vi "Autonomous Independent.vi"() -> ()   [LabVIEW 2016]
doc: "This VI is called when autonomous begins, and will automatically be terminated when autonomous ends. You can carry out timed or sensor driven robot movement independently without needing to return to the caller."
uses:
  2_8_17/Auto_Action.ctl
  <vilib>/Rock Robotics/Network Tables/NT Read Number.vi
  2_11_17/Systems/Global 1.vi
panel:
  out "Terminated?":bool
  out "Auto Mode":dbl=7.0
  in  "Auton_Modes":T2(array[cluster])=[{"Actions"=[{"Effort"=0.55, "Duration"=3.5, "Action"=enum."Nothing", "Encoder"=0.0, "Condition"=FALSE}, {"Effort"=0.0, "Duration"=0.0, "Action"=enum."Nothing", "Encoder"=0.0, "Condition"=FALSE}]}, {"Actions"=[{"Effort"=0.0, "Duration"=0.1, "Action"=enum."Gear1", "Encoder"=6.462, "Condition"=FALSE}, {"Effort"=0.0, "Duration"=0.1, "Action"=enum."Nothing", "Encoder"=0.0, "Condition"=FALSE}, {"Effort"=0.25, "Duration"=1.0, "Action"=enum."Nothing", "Encoder"=38.0, "Condition"=FALSE}, {"Effort"=0.0, "Duration"=0.1, "Action"=enum."Nothing", "Encoder"=0.0, "Condition"=FALSE}, {"Effort"=0.25, "Duration"=0.0, "Action"=enum."Nothing", "Encoder"=57.0, "Condition"=FALSE}, {"Effort"=-0.25, "Duration"=0.0, "Action"=enum."Nothing", "Encoder"=0.0, "Condition"=FALSE}, {"Effort"=1.0, "Duration"=0.0, "Action"=enum."Nothing", "Encoder"=0.0, "Condition"=FALSE}, {"Effort"=0.25, "Duration"=0.0, "Action"=enum."Nothing", "Encoder"=0.0, "Condition"=FALSE}]}, {"Actions"=[{"Effort"=0.0, "Duration"=0.1, "Action"=enum."Drive Encoder Reset", "Encoder"=0.0, "Condition"=FALSE}, {"Effort"=0.0, "Duration"=1.0, "Action"=enum."Gyro Reset", "Encoder"=0.0, "Condition"=FALSE}, {"Effort"=500.0, "Duration"=3.5, "Action"=enum."Drive", "Encoder"=88.0, "Condition"=FALSE}, {"Effort"=1.0, "Duration"=1.0, "Action"=enum."Gear0", "Encoder"=0.0, "Condition"=FALSE}, {"Effort"=1.0, "Duration"=1.0, "Action"=enum."Gear0", "Encoder"=0.0, "Condition"=FALSE}, {"Effort"=1.0, "Duration"=0.5, "Action"=enum."Nothing", "Encoder"=0.0, "Condition"=FALSE}, {"Effort"=0.0, "Duration"=0.0, "Action"=enum."Drive Encoder Reset", "Encoder"=0.0, "Condition"=FALSE}, {"Effort"=500.0, "Duration"=0.5, "Action"=enum."Drive", "Encoder"=24.0, "Condition"=TRUE}, {"Effort"=0.0, "Duration"=0.0, "Action"=enum."Drive Encoder Reset", "Encoder"=0.0, "Condition"=FALSE}, {"Effort"=-500.0, "Duration"=0.0, "Action"=enum."Drive", "Encoder"=24.0, "Condition"=FALSE}, {"Effort"=0.0, "Duration"=0.0, "Action"=enum."Drive Encoder Reset", "Encoder"=0.0, "Condition"=FALSE}, {"Effort"=-0.25, "Duration"=0.0, "Action"=enum."Nothing", "Encoder"=12.0, "Condition"=FALSE}]}, {"Actions"=[{"Effort"=0.0, "Duration"=0.1, "Action"=enum."Drive Encoder Reset", "Encoder"=6.462, "Condition"=FALSE}, {"Effort"=0.0, "Duration"=0.1, "Action"=enum."Gyro Reset", "Encoder"=0.0, "Condition"=FALSE}, {"Effort"=-0.25, "Duration"=1.0, "Action"=enum."Drive", "Encoder"=6.462, "Condition"=FALSE}, {"Effort"=0.0, "Duration"=0.1, "Action"=enum."Gyro Reset", "Encoder"=0.0, "Condition"=FALSE}, {"Effort"=-0.25, "Duration"=0.0, "Action"=enum."Turn", "Encoder"=57.0, "Condition"=FALSE}, {"Effort"=-0.25, "Duration"=0.0, "Action"=enum."Drive", "Encoder"=7.5, "Condition"=FALSE}, {"Effort"=-1.0, "Duration"=0.0, "Action"=enum."Gear0", "Encoder"=0.0, "Condition"=FALSE}, {"Effort"=0.25, "Duration"=0.0, "Action"=enum."Drive", "Encoder"=3.0, "Condition"=FALSE}]}, {"Actions"=[{"Effort"=0.0, "Duration"=0.1, "Action"=enum."Drive Encoder Reset", "Encoder"=6.462, "Condition"=FALSE}, {"Effort"=0.0, "Duration"=0.1, "Action"=enum."Gyro Reset", "Encoder"=0.0, "Condition"=FALSE}, {"Effort"=-0.25, "Duration"=1.0, "Action"=enum."Drive", "Encoder"=6.462, "Condition"=FALSE}, {"Effort"=0.0, "Duration"=0.1, "Action"=enum."Gyro Reset", "Encoder"=0.0, "Condition"=FALSE}, {"Effort"=-0.25, "Duration"=0.0, "Action"=enum."Turn", "Encoder"=57.0, "Condition"=FALSE}, {"Effort"=-0.25, "Duration"=0.0, "Action"=enum."Drive", "Encoder"=7.5, "Condition"=FALSE}, {"Effort"=-1.0, "Duration"=0.0, "Action"=enum."Gear0", "Encoder"=0.0, "Condition"=FALSE}, {"Effort"=0.25, "Duration"=0.0, "Action"=enum."Drive", "Encoder"=3.0, "Condition"=FALSE}]}, {"Actions"=[{"Effort"=0.0, "Duration"=0.1, "Action"=enum."Drive Encoder Reset", "Encoder"=0.0, "Condition"=FALSE}, {"Effort"=0.0, "Duration"=0.1, "Action"=enum."Gyro Reset", "Encoder"=0.0, "Condition"=FALSE}, {"Effort"=0.25, "Duration"=1.0, "Action"=enum."Drive", "Encoder"=6.462, "Condition"=FALSE}, {"Effort"=1.0, "Duration"=0.1, "Action"=enum."Gyro Reset", "Encoder"=0.0, "Condition"=FALSE}, {"Effort"=0.25, "Duration"=0.0, "Action"=enum."Turn", "Encoder"=57.0, "Condition"=FALSE}, {"Effort"=0.25, "Duration"=0.0, "Action"=enum."Drive", "Encoder"=7.5, "Condition"=FALSE}, {"Effort"=1.0, "Duration"=0.0, "Action"=enum."Gear0", "Encoder"=0.0, "Condition"=FALSE}, {"Effort"=-0.25, "Duration"=0.0, "Action"=enum."Drive", "Encoder"=3.0, "Condition"=FALSE}]}, {"Actions"=[{"Effort"=0.0, "Duration"=0.1, "Action"=enum."Drive Encoder Reset", "Encoder"=0.0, "Condition"=FALSE}, {"Effort"=0.0, "Duration"=0.1, "Action"=enum."Gyro Reset", "Encoder"=0.0, "Condition"=FALSE}, {"Effort"=0.25, "Duration"=2.0, "Action"=enum."Drive", "Encoder"=60.0, "Condition"=FALSE}, {"Effort"=0.75, "Duration"=1.0, "Action"=enum."Nothing", "Encoder"=0.0, "Condition"=FALSE}, {"Effort"=0.0, "Duration"=1.0, "Action"=enum."Nothing", "Encoder"=0.0, "Condition"=FALSE}, {"Effort"=0.0, "Duration"=0.0, "Action"=enum."Nothing", "Encoder"=0.0, "Condition"=FALSE}]}, {"Actions"=[{"Effort"=0.0, "Duration"=0.5, "Action"=enum."Drive Encoder Reset", "Encoder"=0.0, "Condition"=FALSE}, {"Effort"=0.55, "Duration"=4.25, "Action"=enum."Gyro Reset", "Encoder"=0.0, "Condition"=FALSE}, {"Effort"=500.0, "Duration"=0.0, "Action"=enum."Drive", "Encoder"=60.0, "Condition"=FALSE}, {"Effort"=0.25, "Duration"=1.4, "Action"=enum."Turn", "Encoder"=0.0, "Condition"=FALSE}, {"Effort"=0.25, "Duration"=2.0, "Action"=enum."Vision Correction", "Encoder"=76.6, "Condition"=FALSE}, {"Effort"=500.0, "Duration"=0.0, "Action"=enum."Drive", "Encoder"=0.0, "Condition"=FALSE}]}, {"Actions"=[{"Effort"=0.0, "Duration"=0.0, "Action"=enum."Nothing", "Encoder"=0.0, "Condition"=FALSE}]}]
  # "Nothing"
  # "Boiler Right Right side gear"
  # "Middle Gear"
  # "Boiler Right Left Side Gear"
  # "Boiler Left RightSide Gear"
  # "Boiler Left Left Side Gear"
  # "Drive"
  # "Vision Correction"
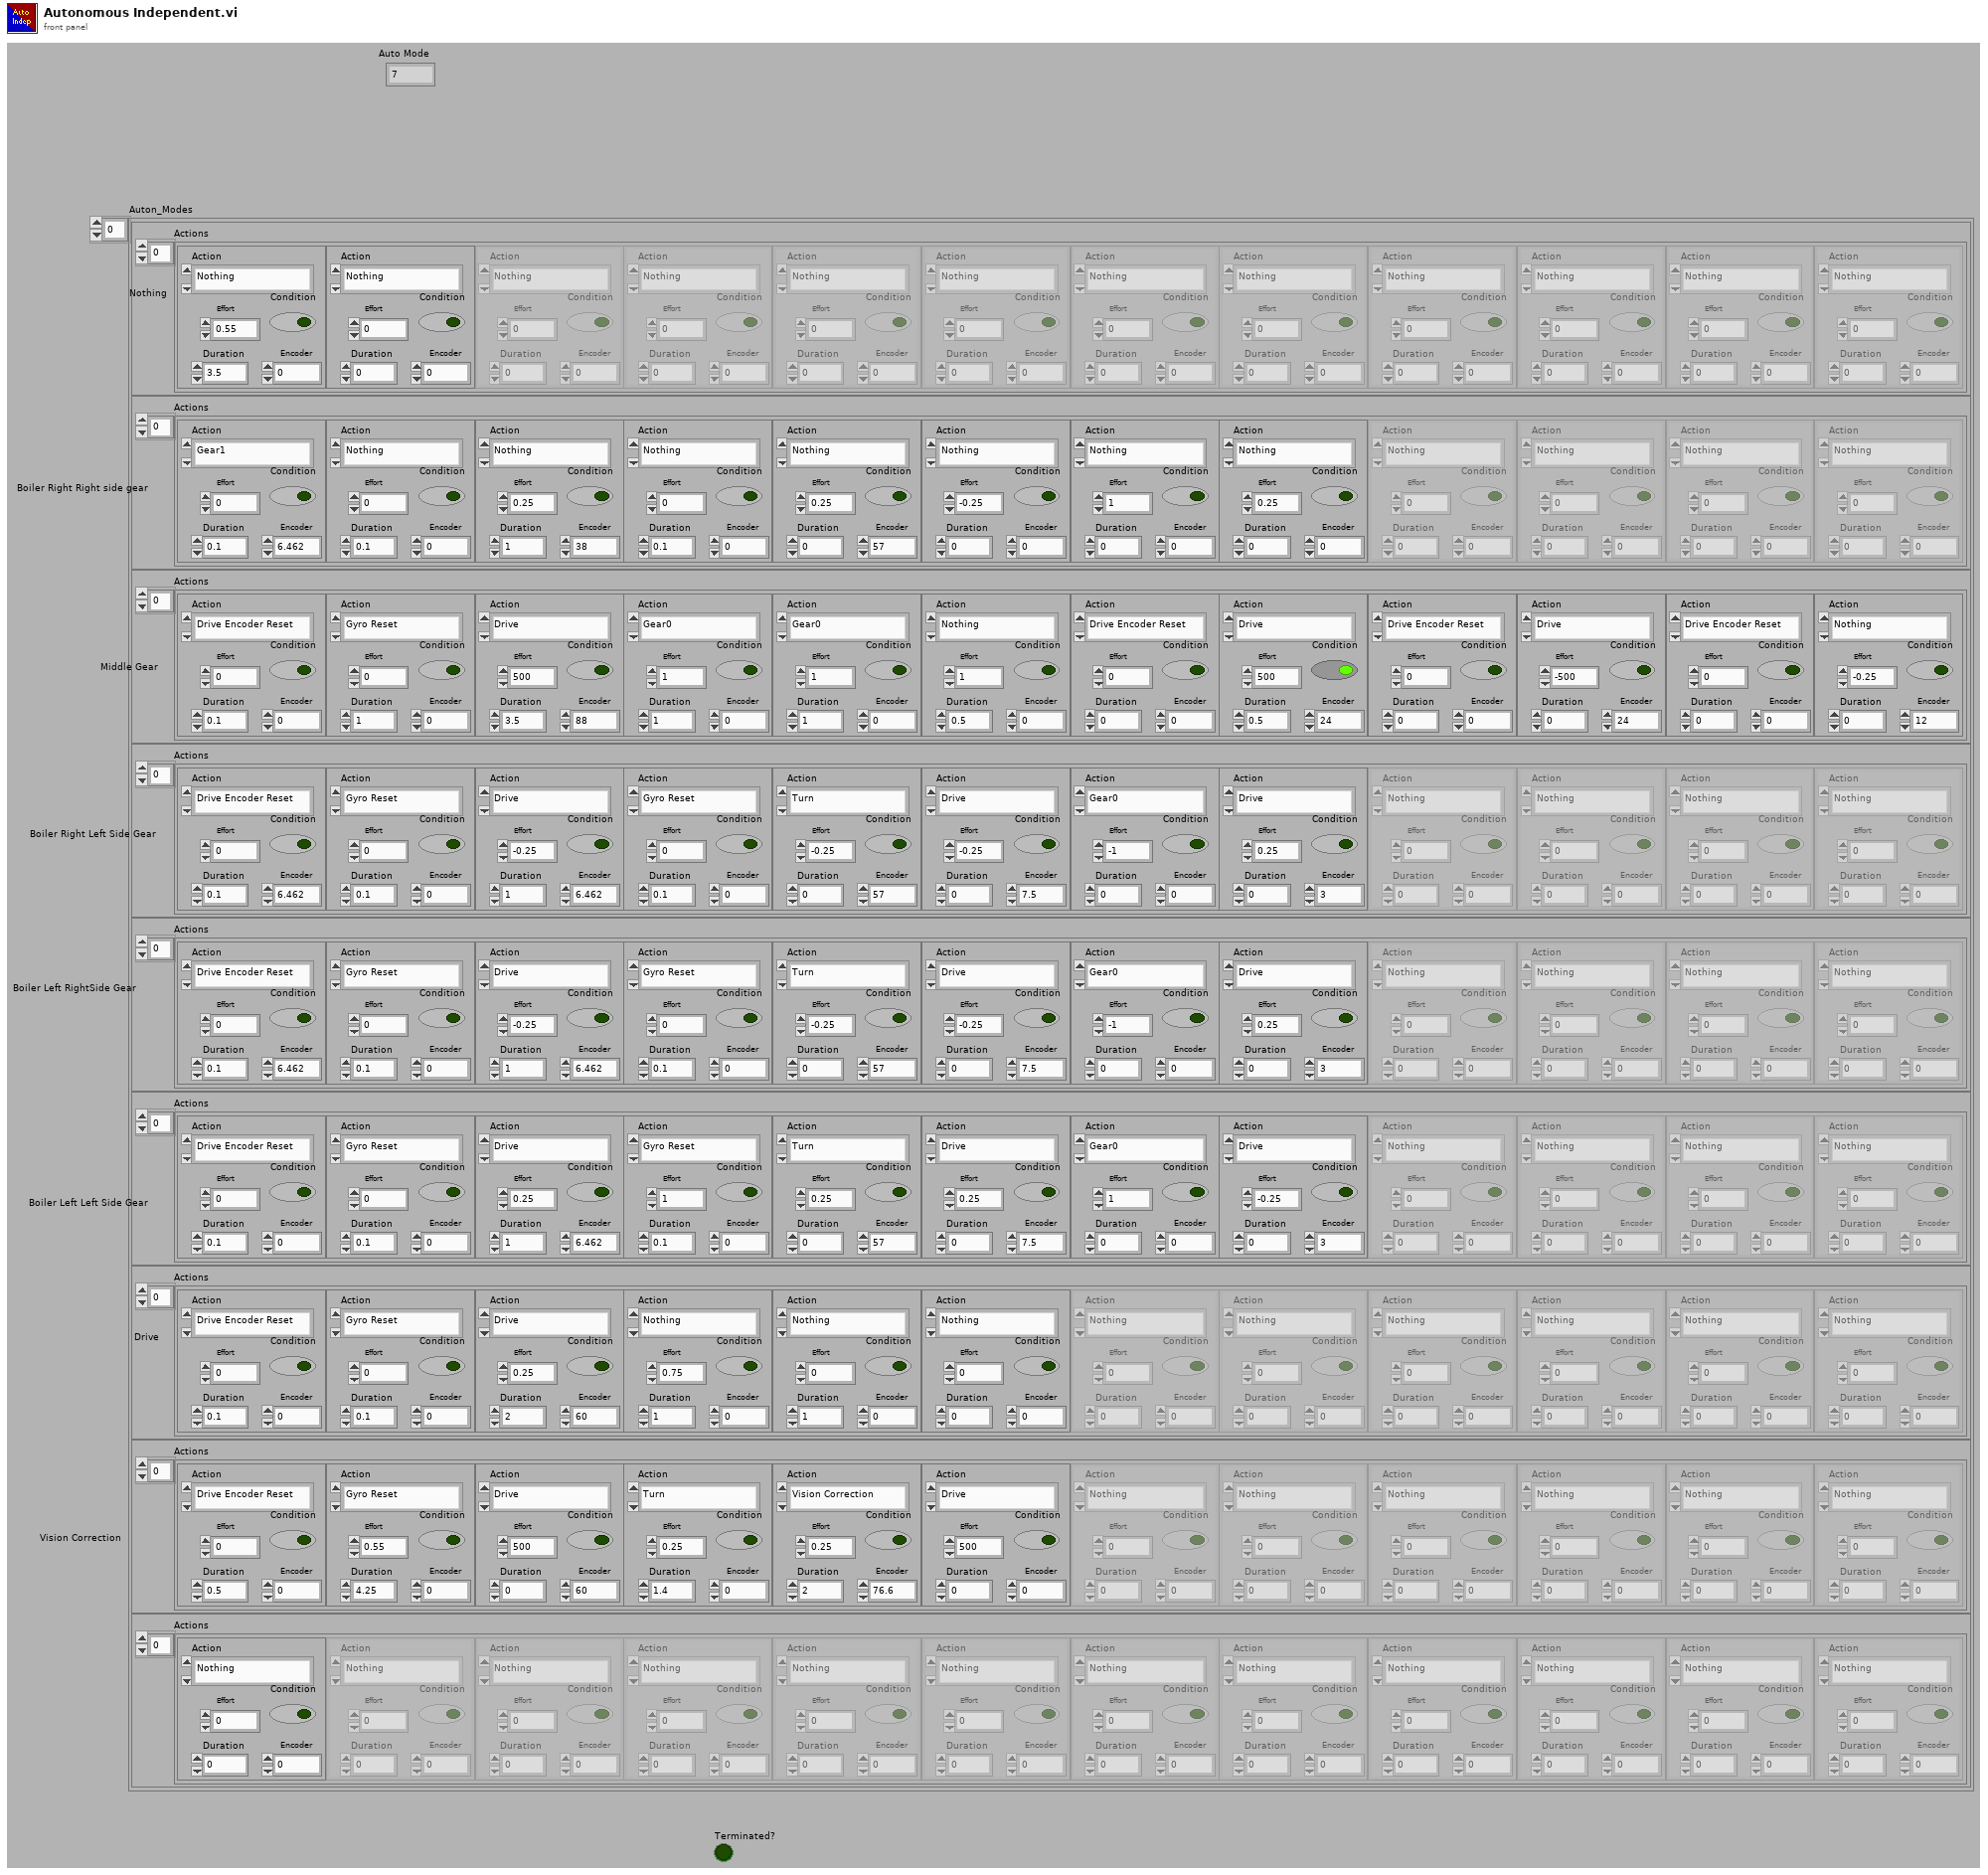
[diagram p1: front panel]
types:
  T1 = typedef "Auto_Action.ctl" = enum16{"Nothing", "Drive", "Vision Correction", "Turn", "Gear0", "Gear1", "Climb", "Intake", "Index", "Shoot", "Test", "Drive Encoder Reset", "Gyro Reset"}
  T2 = cluster{"Actions":cluster{"Effort":dbl, "Duration":dbl, "Action":T1, "Encoder":dbl, "Condition":bool}[]}[]
  T3 = cluster{"Actions":cluster{"Effort":dbl, "Duration":dbl, "Action":T1, "Encoder":dbl, "Condition":bool}[]}
  T4 = cluster{"Effort":dbl, "Duration":dbl, "Action":T1, "Encoder":dbl, "Condition":bool}[]
  T5 = typedef "WPI_MotorControlDeviceRef.ctl" = cluster{"DeviceStatus":errorcluster, "Type":T6, "PWM":cluster{"PWM Channel":T7, "DeadBand":T8}, "CAN":cluster{"Device Number":u8, "SetOutput VI Ref":variant, "GetOutput VI Ref":variant, "Enable VI Ref":variant, "Disable VI Ref":variant, "Data":variant}, "Invert":bool}
  T6 = typedef "WPI_MotorControlType.ctl" = enum16{"PWM", "CAN"}
  T7 = typedef "FPGA_DIOPWMChannel.ctl" = enum8{"PWM 0", "PWM 1", "PWM 2", "PWM 3", "PWM 4", "PWM 5", "PWM 6", "PWM 7", "PWM 8", "PWM 9", "PWM MXP 0", "PWM MXP 1", "PWM MXP 2", "PWM MXP 3", "PWM MXP 4", "PWM MXP 5", "PWM MXP 6", "PWM MXP 7", "PWM MXP 8", "PWM MXP 9", "Invalid"}
  T8 = typedef "WPI_PWMDeadband.ctl" = cluster{"Name":string, "maxPositivePwm":i32, "minPositivePwm":i32, "centerPwm":i32, "maxNegativePwm":i32, "minNegativePwm":i32, "angularRange":u16}
  T9 = typedef "WPI_CANTalonSRX_GlobalStatus.ctl" = cluster{"Applied Throttle":dbl, "Module Enabled":bool, "CAN Error":errorcluster, "Closed Loop Error":dbl, "Forward Limit Switch Closed":bool, "Reverse Limit Switch Closed":bool, "Sensor Position":dbl, "Sensor Velocity":dbl, "Current":dbl, "Sticky Fault - Over Temp":bool, "Sticky Fault - Under Voltage":bool, "Sticky Fault - Forward Limit":bool, "Sticky Fault - Reverse Limit":bool, "Sticky Fault - Forward Soft Limit":bool, "Sticky Fault - Reverse Soft Limit":bool, "Brake is Enabled":bool, "Encoder Position":dbl, "Encoder Velocity":dbl, "Encoder Index Count":dbl, "Encoder A Pin State":bool, "Encoder B Pin State":bool, "Encoder Index Pin State":bool, "Analog In":dbl, "Analog In Velocity":dbl, "Temperature (C)":dbl, "Battery Voltage":dbl, "Control 5 Is Supported":bool, "Current Profile Slot Select":dbl, "Pos Div 8":bool, "Vel Div 4":bool, "Pulse Width Position":i32, "Pulse Width Velocity":i32, "Pulse Width Rise To Rise (us)":i32, "Pulse Width Rise To Fall (us)":i32, "Mot Prof Active Is Under Run":bool, "Mot Prof Active Has Under Run":bool, "Mot Prof Active Is Last":bool, "Mot Prof Active Velocity Only":bool, "Mot Prof Active Is Valid":bool, "Mot Prof Buffer Is Full":bool, "Mot Prof Active Profile Slot Select":i32, "Mot Prof NextID":i32, "Mot Prof Count":i32, "Mot Prof Active Velocity":dbl, "Mot Prof Active Position":dbl, "Mot Prof Output Enable":i32}
  T10 = typedef "WPI_GyroDevRef.ctl" = cluster{"DevStatus":errorcluster, "Analog Channel":T11, "Offset":dbl, "Gain (VoltsPerDegree/Second)":dbl, "Gyro Type":enum16{"Analog", "XRS450"}, "Handle":i32, "SPI Bus":T12, "Device Found":bool, "Sample Rate":dbl, "Calibrate On Open":bool}
  T11 = typedef "FPGA_AIChannel.ctl" = enum8{"AI 0", "AI 1", "AI 2", "AI 3", "AI MXP 0", "AI MXP 1", "AI MXP 2", "AI MXP 3", "Invalid"}
  T12 = typedef "spi_bus.ctl" = enum16{"SPI On-Board, CS0", "SPI On-Board, CS1", "SPI On-Board, CS2", "SPI On-Board, CS3", "SPI MXP", "Invalid"}
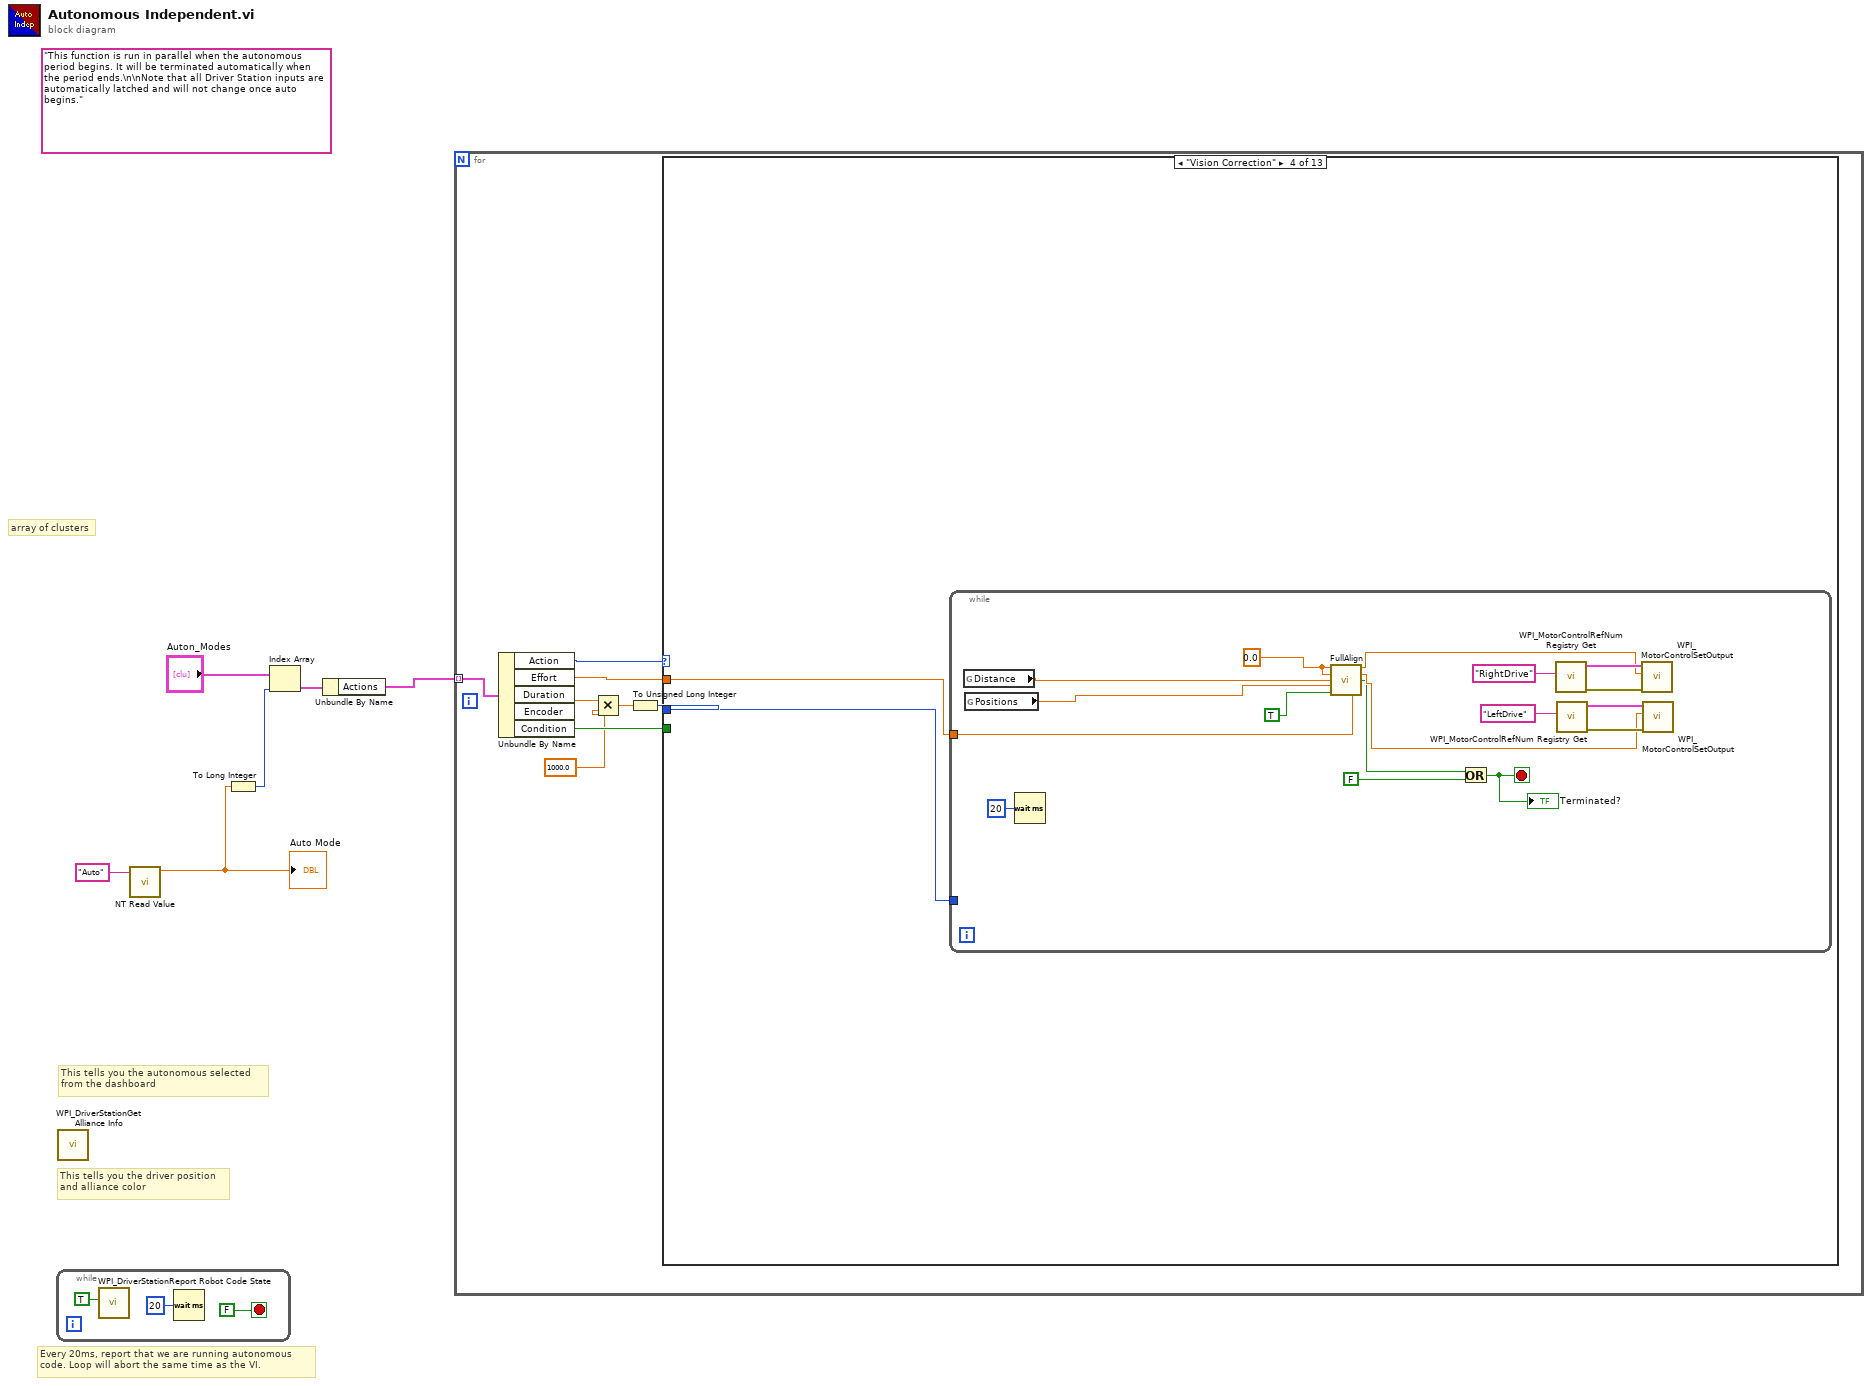
[diagram p0: block diagram]
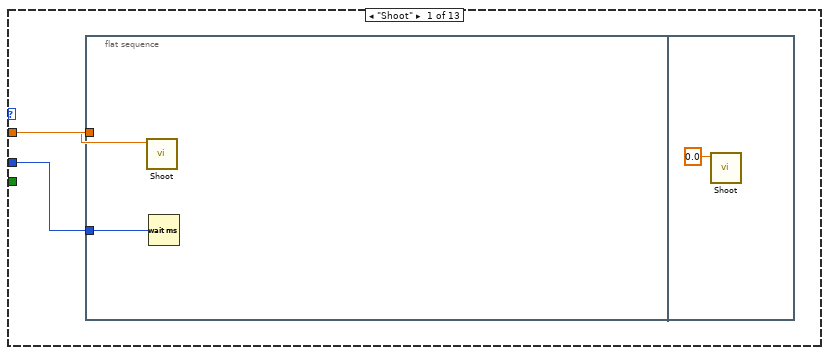
[diagram p2: hidden frame]
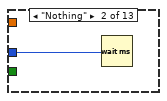
[diagram p3: hidden frame]
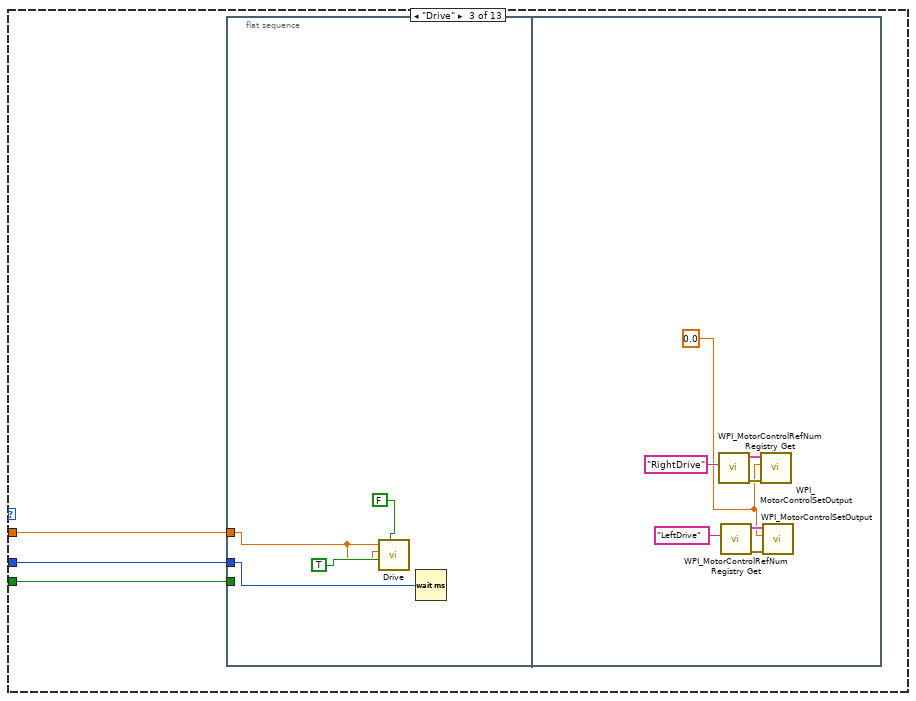
[diagram p4: hidden frame]
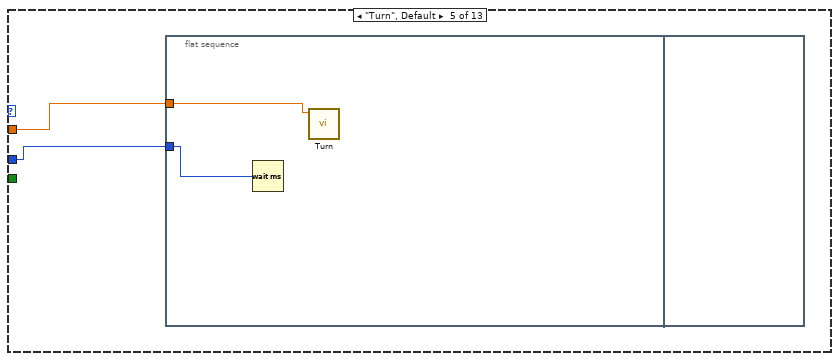
[diagram p5: hidden frame]
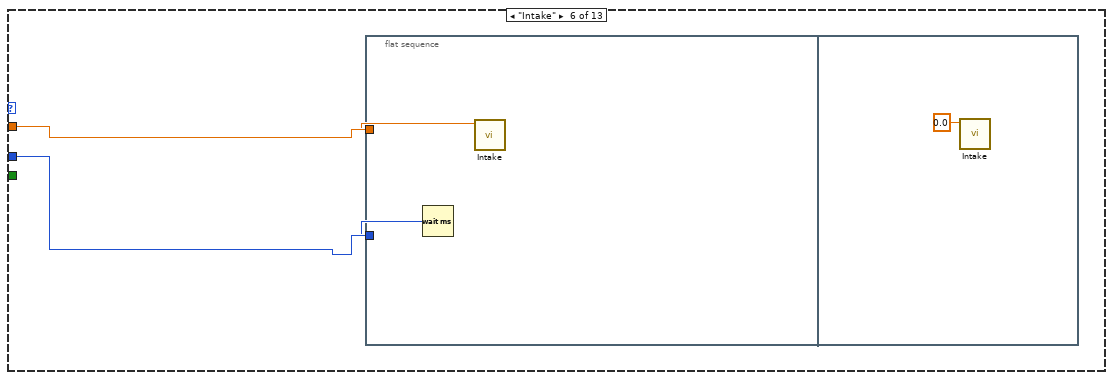
[diagram p6: hidden frame]
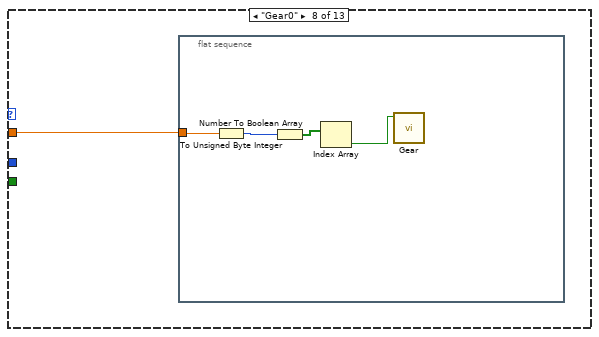
[diagram p8: hidden frame]
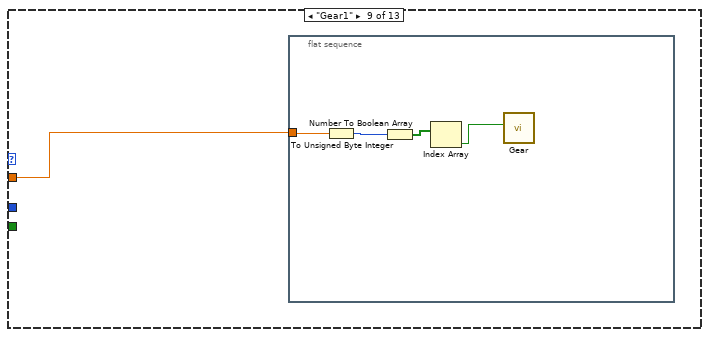
[diagram p9: hidden frame]
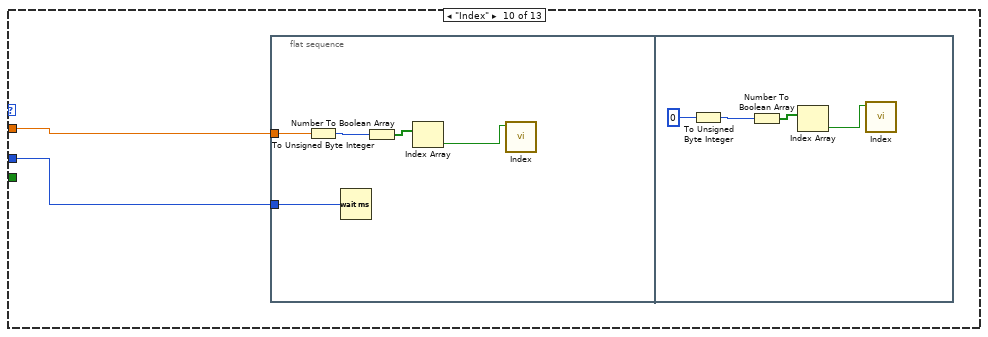
[diagram p10: hidden frame]
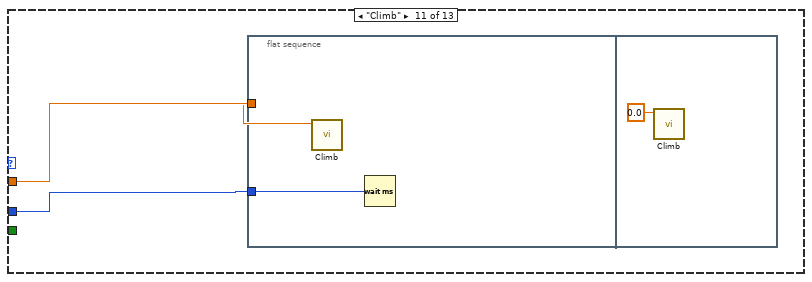
[diagram p11: hidden frame]
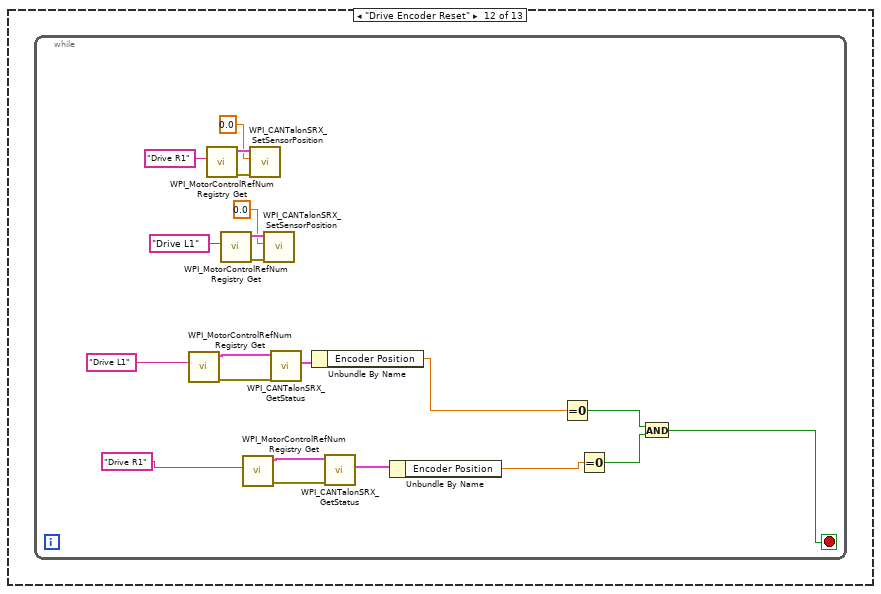
[diagram p12: hidden frame]
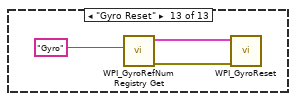
[diagram p13: hidden frame]
diagram:
  (unwired) "This function is run in parallel when the autonomous period begins. It will be terminated automatically when the period ends.\n\nNote that all Driver Station inputs are automatically latched and will not change once auto begins."
  # "This tells you the autonomous selected\nfrom the dashboard"
  # "array of clusters"
  # "Every 20ms, report that we are running autonomous\ncode. Loop will abort the same time as the VI."
  # "This tells you the driver position\nand alliance color"
  n1 = while {
    stop <- FALSE stop-if-true
    n2 = call <vilib>:"WPI_DriverStationReport Robot Code State.vi"("Autonomous"=TRUE) -> ()  [unwired: 10 in, 1 out]
    n3 = Wait (ms)(milliseconds to wait=u32 20) -> ()  [unwired: 1 out]
  }
  n4 = call <vilib>:"WPI_DriverStationGet Alliance Info.vi"() -> ()  [unwired: 12 out]
  n5 = call-poly <vilib>:"NT Read Value.vi"("Name"="Auto") -> ("Numeric"=w1:dbl)  [unwired: 9 in, 1 out]
  "Auto Mode" <- w1
  n6 = To Long Integer(number=w1) -> (32bit integer=w3:i32)
  n7 = Index Array(array="Auton_Modes", index=w3) -> (element=w5:T3)
  n8 = Unbundle By Name(w5) -> ("Actions"=w6:T4)
  n9 = for {
    tunnel: w6 -> [w17] mode=indexing
    n10 = Unbundle By Name(w17) -> ("Action"=w16:T1, "Effort"=w15:dbl, "Duration"=w14:dbl, "Condition"=w11:bool)  [unwired: 1 out]
    n11 = Multiply(x=w14, y=1000.0) -> (x*y=w13:dbl)
    n12 = To Unsigned Long Integer(number=w13) -> (unsigned 32bit integer=w12:u32)
    n13 = case shown="\"Vision Correction\"" w16 {
      tunnel: w15 -> [w19 _ w26 w38 w58 w62 _ w66 w71 w76 w88 _ _]
      tunnel: w12 -> [w18 w23 w25 w39 w57 w61 _ _ _ w77 w87 _ _]
      tunnel: w11 -> [_ _ w24 _ _ _ _ _ _ _ _ _ _]
      frame "Shoot" {
        n14 = flat-sequence {
          tunnel: w19 -> [w21]
          tunnel: w18 -> [w20]
          frame #0 {
            n15 = call "Shoot.vi"("Set RPM"=w21) -> ()  [unwired: 11 in]
            n16 = Wait (ms)(milliseconds to wait=w20) -> ()  [unwired: 1 out]
          }
          frame #1 {
            n17 = call "Shoot.vi"("Set RPM"=0.0 ("Effort")) -> ()  [unwired: 11 in]
          }
        }
      }
      frame "Nothing" {
        n18 = Wait (ms)(milliseconds to wait=w23) -> ()  [unwired: 1 out]
      }
      frame "Drive" {
        n19 = flat-sequence {
          tunnel: w26 -> [w27]
          tunnel: w25 -> [w30]
          tunnel: w24 -> [_]
          frame #0 {
            n20 = call "Drive.vi"("Slow?"=FALSE, "SwitchDir"=TRUE, "Drive L"=w27, "Drive R"=w27) -> ()  [unwired: 8 in]
            n21 = Wait (ms)(milliseconds to wait=w30) -> ()  [unwired: 1 out]
          }
          frame #1 {
            w31 = 0.0
            n22 = call <vilib>:"WPI_MotorControlRefNum Registry Get.vi"("refnum name"="RightDrive") -> ("error out"=w34:errorcluster, "MotorControlDevRef"=w32:T5)  [unwired: 9 in]
            n23 = call <vilib>:"WPI_MotorControlRefNum Registry Get.vi"("refnum name"="LeftDrive") -> ("error out"=w35:errorcluster, "MotorControlDevRef"=w36:T5)  [unwired: 9 in]
            n24 = call <vilib>:"WPI_MotorControlSetOutput.vi"("error in (no error)"=w34, "Output"=w31, "MotorControlDevRef"=w32) -> ()  [unwired: 6 in, 3 out]
            n25 = call <vilib>:"WPI_MotorControlSetOutput.vi"("error in (no error)"=w35, "Output"=w31, "MotorControlDevRef"=w36) -> ()  [unwired: 6 in, 3 out]
          }
        }
      }
      frame "Vision Correction" {
        n26 = while {
          tunnel: w39 -> [_]
          tunnel: w38 -> [w40]
          stop <- w44 stop-if-true
          w48 = 0.0
          n27 = global read "Global 1.vi" "Distance"() -> (w46:dbl)
          n28 = global read "Global 1.vi" "Positions"() -> (w45:dbl)
          n29 = Wait (ms)(milliseconds to wait=u32 20) -> ()  [unwired: 1 out]
          n30 = call "FullAlign.vi"("Joystick 0"=w48, "Joystick 1"=w48, "Distance"=w46, "Angle"=w45, "Button"=TRUE, "Effort"=w40) -> ("Right Motor"=w50:dbl, "Left Motor"=w49:dbl, "In Range?"=w42:bool)  [unwired: 6 in, 1 out]
          n31 = Or(x=w42, y=FALSE) -> (x .or. y?=w44:bool)
          "Terminated?" <- w44
          n32 = call <vilib>:"WPI_MotorControlRefNum Registry Get.vi"("refnum name"="RightDrive") -> ("error out"=w51:errorcluster, "MotorControlDevRef"=w53:T5)  [unwired: 9 in]
          n33 = call <vilib>:"WPI_MotorControlRefNum Registry Get.vi"("refnum name"="LeftDrive") -> ("error out"=w54:errorcluster, "MotorControlDevRef"=w55:T5)  [unwired: 9 in]
          n34 = call <vilib>:"WPI_MotorControlSetOutput.vi"("error in (no error)"=w51, "Output"=w50, "MotorControlDevRef"=w53) -> ()  [unwired: 6 in, 3 out]
          n35 = call <vilib>:"WPI_MotorControlSetOutput.vi"("error in (no error)"=w54, "Output"=w49, "MotorControlDevRef"=w55) -> ()  [unwired: 6 in, 3 out]
        }
      }
      frame "Turn", Default {
        n36 = flat-sequence {
          tunnel: w58 -> [w60]
          tunnel: w57 -> [w59]
          frame #0 {
            n37 = Wait (ms)(milliseconds to wait=w59) -> ()  [unwired: 1 out]
            n38 = call "Turn.vi"("Effort"=w60) -> ()  [unwired: 11 in]
          }
          frame #1 {
          }
        }
      }
      frame "Intake" {
        n39 = flat-sequence {
          tunnel: w62 -> [w64]
          tunnel: w61 -> [w63]
          frame #0 {
            n40 = Wait (ms)(milliseconds to wait=w63) -> ()  [unwired: 1 out]
            n41 = call "Intake.vi"("Effort"=w64) -> ()  [unwired: 11 in]
          }
          frame #1 {
            n42 = call "Intake.vi"("Effort"=0.0) -> ()  [unwired: 11 in]
          }
        }
      }
      frame "Test" {
      }
      frame "Gear0" {
        n43 = flat-sequence {
          tunnel: w66 -> [w70]
          frame #0 {
            n44 = To Unsigned Byte Integer(number=w70) -> (unsigned 8bit integer=w69:u8)
            n45 = Number To Boolean Array(number=w69) -> (Boolean array=w68:bool[])
            n46 = Index Array(array=w68) -> (element=w67:bool)  [unwired: 1 in]
            n47 = call "Gear.vi"("Gear0?"=w67) -> ()  [unwired: 11 in]
          }
        }
      }
      frame "Gear1" {
        n48 = flat-sequence {
          tunnel: w71 -> [w75]
          frame #0 {
            n49 = To Unsigned Byte Integer(number=w75) -> (unsigned 8bit integer=w74:u8)
            n50 = Number To Boolean Array(number=w74) -> (Boolean array=w73:bool[])
            n51 = Index Array(array=w73) -> (element=w72:bool)  [unwired: 1 in]
            n52 = call "Gear.vi"("Gear1?"=w72) -> ()  [unwired: 11 in]
          }
        }
      }
      frame "Index" {
        n53 = flat-sequence {
          tunnel: w77 -> [w79]
          tunnel: w76 -> [w78]
          frame #0 {
            n54 = To Unsigned Byte Integer(number=w78) -> (unsigned 8bit integer=w82:u8)
            n55 = Wait (ms)(milliseconds to wait=w79) -> ()  [unwired: 1 out]
            n56 = Number To Boolean Array(number=w82) -> (Boolean array=w81:bool[])
            n57 = Index Array(array=w81) -> (element=w80:bool)  [unwired: 1 in]
            n58 = call "Index.vi"("Index?"=w80) -> ()  [unwired: 11 in]
          }
          frame #1 {
            n59 = To Unsigned Byte Integer(number=u8 0) -> (unsigned 8bit integer=w85:u8)
            n60 = Number To Boolean Array(number=w85) -> (Boolean array=w86:bool[])
            n61 = Index Array(array=w86) -> (element=w83:bool)  [unwired: 1 in]
            n62 = call "Index.vi"("Index?"=w83) -> ()  [unwired: 11 in]
          }
        }
      }
      frame "Climb" {
        n63 = flat-sequence {
          tunnel: w88 -> [w90]
          tunnel: w87 -> [w89]
          frame #0 {
            n64 = call "Climb.vi"("Effort"=w90) -> ()  [unwired: 11 in]
            n65 = Wait (ms)(milliseconds to wait=w89) -> ()  [unwired: 1 out]
          }
          frame #1 {
            n66 = call "Climb.vi"("Effort"=0.0) -> ()  [unwired: 11 in]
          }
        }
      }
      frame "Drive Encoder Reset" {
        n67 = while {
          stop <- w92 stop-if-true
          n68 = call <vilib>:"WPI_MotorControlRefNum Registry Get.vi"("refnum name"="Drive L1") -> ("error out"=w102:errorcluster, "MotorControlDevRef"=w97:T5)  [unwired: 9 in]
          n69 = call <vilib>:"WPI_MotorControlRefNum Registry Get.vi"("refnum name"="Drive R1") -> ("error out"=w107:errorcluster, "MotorControlDevRef"=w106:T5)  [unwired: 9 in]
          n70 = call <vilib>:"WPI_MotorControlRefNum Registry Get.vi"("refnum name"="Drive L1") -> ("error out"=w109:errorcluster, "MotorControlDevRef"=w110:T5)  [unwired: 9 in]
          n71 = call <vilib>:"WPI_MotorControlRefNum Registry Get.vi"("refnum name"="Drive R1") -> ("error out"=w99:errorcluster, "MotorControlDevRef"=w98:T5)  [unwired: 9 in]
          n72 = call <vilib>:"WPI_CANTalonSRX_SetSensorPosition.vi"("error in (no error)"=w107, "New Sensor Position"=0.0, "CAN Talon SRX Ref"=w106) -> ()  [unwired: 7 in, 2 out]
          n73 = call <vilib>:"WPI_CANTalonSRX_SetSensorPosition.vi"("error in (no error)"=w109, "New Sensor Position"=0.0, "CAN Talon SRX Ref"=w110) -> ()  [unwired: 7 in, 2 out]
          n74 = call <vilib>:"WPI_CANTalonSRX_GetStatus.vi"("error in (no error)"=w102, "CAN Talon SRX Ref"=w97) -> ("Talon SRX Status"=w100:T9)  [unwired: 7 in, 2 out]
          n75 = Unbundle By Name(w100) -> ("Encoder Position"=w95:dbl)
          n76 = call <vilib>:"WPI_CANTalonSRX_GetStatus.vi"("error in (no error)"=w99, "CAN Talon SRX Ref"=w98) -> ("Talon SRX Status"=w101:T9)  [unwired: 7 in, 2 out]
          n77 = Unbundle By Name(w101) -> ("Encoder Position"=w96:dbl)
          n78 = Equal To 0?(x=w95) -> (x = 0?=w94:bool)
          n79 = Equal To 0?(x=w96) -> (x = 0?=w93:bool)
          n80 = And(x=w94, y=w93) -> (x .and. y?=w92:bool)
        }
      }
      frame "Gyro Reset" {
        n81 = call <vilib>:"WPI_GyroRefNum Registry Get.vi"("refnum name"="Gyro") -> ("error out"=w114:errorcluster, "GyroDevRef"=w115:T10)  [unwired: 9 in]
        n82 = call <vilib>:"WPI_GyroReset.vi"("error in"=w114, "GyroDevRef"=w115) -> ()  [unwired: 8 in, 2 out]
      }
    }
  }
